vi "Read 1st M y ref.vi"(8 "error in (no error)":errorcluster, 11 "Analyze Results Second Momentum in":refnum<class "Analyze Results Second Momentum.lvclass">) -> (0 "error out":errorcluster, 2 "1st M y ref":refnum<vi>, 3 "Analyze Results Second Momentum out":refnum<class "Analyze Results Second Momentum.lvclass">)   [LabVIEW 2014, in "Analyze Results Second Momentum.lvclass"]
uses:
  Analyze Results Second Momentum.lvclass
  Analyze Results Second Momentum.lvclass/Analyze Results Second Momentum.ctl
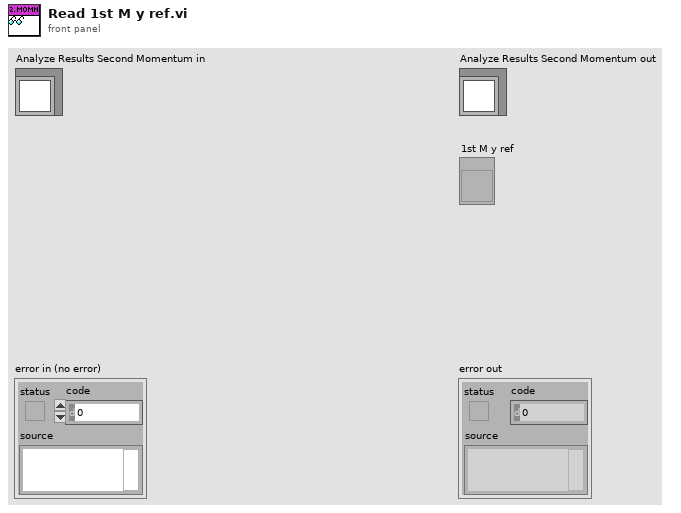
[diagram p1: front panel]
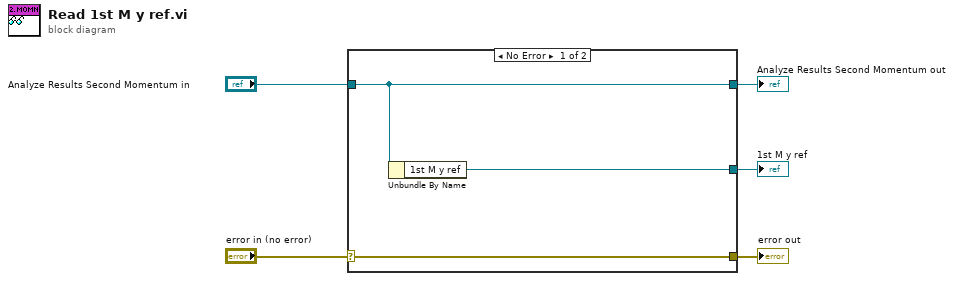
[diagram p0: block diagram]
diagram:
  n1 = case shown="No Error" "error in (no error)" {
    selector: "error in (no error)" -> [w8 w9]
    tunnel: [w8 w9] -> w4
    tunnel: [w7 w10] -> w2
    tunnel: "Analyze Results Second Momentum in" -> [w7 w10]
    tunnel: [w6 _] -> w1
    frame No Error {
      n2 = Unbundle By Name(w7) -> ("1st M y ref"=w6:refnum<vi>)
    }
    frame Error {
    }
  }
  "error out" <- w4
  "Analyze Results Second Momentum out" <- w2
  "1st M y ref" <- w1
